vi "MGI Bezier Downhill Simplex nD Inner Part.vi"(3 "Iterations":i32, 4 "f(Minimum) Before[]":dbl[](array[numeric]) format="%.2f", 5 "Minimum Before[][]":dbl[][](array[numeric]) format="%.2f") -> (0 "Accuracy":dbl format="%.2f", 1 "f(Minimum) After[]":dbl[](array[numeric]) format="%.2f", 2 "Minimum After[][]":dbl[][](array[numeric]) format="%.2f")   [LabVIEW 2016]
doc: "Modification of nD Simplex routine provided with LabVIEW. At each iteration, this version has a specific calculation hard-coded. Also modified to perform n iterations instead of running until an accuracy spec is met.\n\nAuthored by David A. Moore\nsupport@mooregoodideas.com\nwww.mooregoodideas.com\n\nCopyright (c) 2010, Moore Good Ideas, Inc.\n\nAll rights reserved.\n\nRedistribution and use in source and binary forms, with or without modification, are permitted provided that the following conditions are met:\n\n * Redistributions of source code must retain the above copyright notice, this list of conditions and the following disclaimer.\n * Redistributions in binary form must reproduce the above copyright notice, this list of conditions and the following disclaimer in the documentation and/or other materials provided with the distribution.\n * Neither the name of Moore Good Ideas, Inc. nor the names of its contributors may be used to endorse or promote products derived from this software without specific prior written permission.\n\nTHIS SOFTWARE IS PROVIDED BY THE COPYRIGHT HOLDERS AND CONTRIBUTORS \"AS IS\" AND ANY EXPRESS OR IMPLIED WARRANTIES, INCLUDING, BUT NOT LIMITED TO, THE IMPLIED WARRANTIES OF MERCHANTABILITY AND FITNESS FOR A PARTICULAR PURPOSE ARE DISCLAIMED. IN NO EVENT SHALL THE COPYRIGHT OWNER OR CONTRIBUTORS BE LIABLE FOR ANY DIRECT, INDIRECT, INCIDENTAL, SPECIAL, EXEMPLARY, OR CONSEQUENTIAL DAMAGES (INCLUDING, BUT NOT LIMITED TO, PROCUREMENT OF SUBSTITUTE GOODS OR SERVICES; LOSS OF USE, DATA, OR PROFITS; OR BUSINESS INTERRUPTION) HOWEVER CAUSED AND ON ANY THEORY OF LIABILITY, WHETHER IN CONTRACT, STRICT LIABILITY, OR TORT (INCLUDING NEGLIGENCE OR OTHERWISE) ARISING IN ANY WAY OUT OF THE USE OF THIS SOFTWARE, EVEN IF ADVISED OF THE POSSIBILITY OF SUCH DAMAGE."
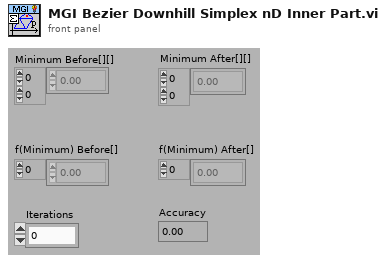
[diagram p1: front panel]
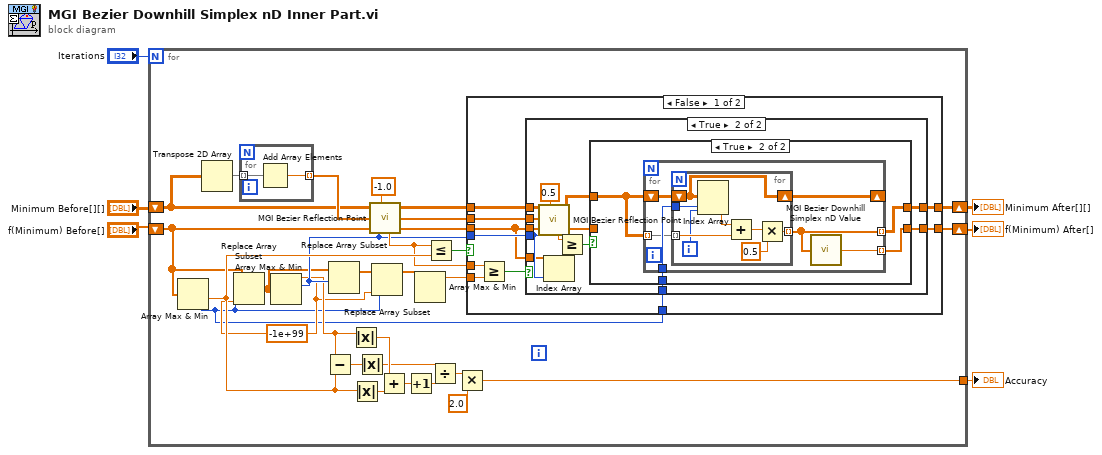
[diagram p0: block diagram]
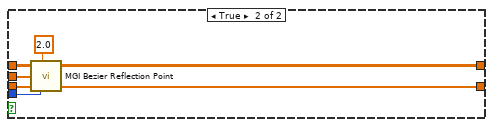
[diagram p4: hidden frame]
diagram:
  n1 = for {
    N: "Iterations" -> [_]
    shift-right: [w10] -> w3
    shift-left: "Minimum Before[][]" -> [w8]
    shift-right: [w9] -> w5
    shift-left: "f(Minimum) Before[]" -> [w15]
    tunnel: [w7] -> w2
    w13 = -1e+99
    n2 = Array Max & Min(array=w15) -> (min value=w28:dbl, min index (indices)=w12:i32)  [unwired: 2 out]
    n3 = Transpose 2D Array(2D array=w8) -> (transposed array=w36:dbl[][])
    n4 = Replace Array Subset(array=w15, new element=w13, index=w12) -> (w14:dbl[])
    n5 = for {
      tunnel: w36 -> [w91] mode=indexing
      tunnel: [w90] -> w25 mode=indexing
      n6 = Add Array Elements(numeric array=w91) -> (sum=w90:dbl)
    }
    n7 = Array Max & Min(array=w14) -> (max value=w16:dbl, max index (indices)=w17:i32)  [unwired: 2 out]
    n8 = Subtract(x=w16, y=w28) -> (x-y=w35:dbl)
    n9 = Replace Array Subset(array=w14, new element=w13, index=w17) -> (w19:dbl[])
    n10 = Absolute Value(x=w16) -> (abs(x)=w34:dbl)
    n11 = Absolute Value(x=w28) -> (abs(x)=w33:dbl)
    n12 = Absolute Value(x=w35) -> (abs(x)=w32:dbl)
    n13 = call <userlib>:"MGI Bezier Reflection Point.vi"("Points Before[][]"=w8, "Factor"=-1.0, "psum Before[]"=w25, "f Values Before[]"=w15, "High Index"=w17) -> ("Points After[][]"=w24:dbl[][], "psum After[]"=w23:dbl[], "New f Value"=w21:dbl, "f Values After[]"=w22:dbl[])  [unwired: 1 in]
    n14 = Replace Array Subset(array=w19, new element=w13, index=w12) -> (w18:dbl[])
    n15 = Add(x=w34, y=w33) -> (x+y=w31:dbl)
    n16 = Increment(x=w31) -> (x+1=w11:dbl)
    n17 = Array Max & Min(array=w18) -> (max value=w20:dbl)  [unwired: 3 out]
    n18 = Less Or Equal?(x=w21, y=w28) -> (x <= y?=w27:bool)
    n19 = Divide(x=w32, y=w11) -> (x/y=w30:dbl)
    n20 = Multiply(x=w30, y=2.0) -> (x*y=w7:dbl)
    n21 = case shown="False" w27 {
      tunnel: w24 -> [w43 w88]
      tunnel: w23 -> [w42 w87]
      tunnel: w22 -> [w37 w86]
      tunnel: w17 -> [w41 w85]
      tunnel: [w39 w84] -> w10
      tunnel: [w38 w83] -> w9
      tunnel: w21 -> [w46 _]
      tunnel: w20 -> [w45 _]
      tunnel: w12 -> [w40 _]
      frame False {
        n22 = Greater Or Equal?(x=w46, y=w45) -> (x >= y?=w44:bool)
        n23 = case shown="True" w44 {
          tunnel: w43 -> [w48 w61]
          tunnel: w42 -> [_ w60]
          tunnel: w37 -> [w47 w59]
          tunnel: w41 -> [_ w51]
          tunnel: w40 -> [_ w56]
          tunnel: [w48 w54] -> w39
          tunnel: [w47 w53] -> w38
          tunnel: w37 -> [_ w50]
          frame False {
          }
          frame True {
            n24 = call <userlib>:"MGI Bezier Reflection Point.vi"("Points Before[][]"=w61, "Factor"=0.5, "psum Before[]"=w60, "f Values Before[]"=w59, "High Index"=w51) -> ("Points After[][]"=w55:dbl[][], "New f Value"=w58:dbl, "f Values After[]"=w52:dbl[])  [unwired: 1 in, 1 out]
            n25 = Index Array(array=w50, index=w51) -> (element=w49:dbl)
            n26 = Greater Or Equal?(x=w58, y=w49) -> (x >= y?=w57:bool)
            n27 = case shown="True" w57 {
              tunnel: w56 -> [_ w68]
              tunnel: w55 -> [w64 w65]
              tunnel: [w64 w67] -> w54
              tunnel: [w63 w66] -> w53
              tunnel: w52 -> [w63 _]
              frame False {
              }
              frame True {
                n28 = for {
                  tunnel: w68 -> [w72]
                  shift-right: [w73] -> _
                  shift-left: w65 -> [w74]
                  tunnel: w65 -> [w71] mode=indexing
                  tunnel: [w70] -> w67 mode=indexing
                  tunnel: [w69] -> w66 mode=indexing
                  n29 = for {
                    shift-right: [w77] -> w73
                    shift-left: w74 -> [w77]
                    tunnel: w72 -> [w75]
                    tunnel: w71 -> [w82] mode=indexing
                    tunnel: [w78] -> w70 mode=indexing
                    i -> [w76]
                    n30 = Index Array(array=w77, index (row)=w75, index (col)=w76) -> (element=w81:dbl)
                    n31 = Add(x=w81, y=w82) -> (x+y=w80:dbl)
                    n32 = Multiply(x=w80, y=0.5) -> (x*y=w78:dbl)
                  }
                  n33 = call <userlib>:"MGI Bezier Downhill Simplex nD Value.vi"("x[]"=w70) -> ("f(x)"=w69:dbl)
                }
              }
            }
          }
        }
      }
      frame True {
        n34 = call <userlib>:"MGI Bezier Reflection Point.vi"("Points Before[][]"=w88, "Factor"=2.0, "psum Before[]"=w87, "f Values Before[]"=w86, "High Index"=w85) -> ("Points After[][]"=w84:dbl[][], "f Values After[]"=w83:dbl[])  [unwired: 1 in, 2 out]
      }
    }
  }
  "f(Minimum) After[]" <- w5
  "Minimum After[][]" <- w3
  "Accuracy" <- w2
